vi "Measure H3611i Range.vi"(8 "error in (no error)":errorcluster, 11 "H3611i Actor in":refnum<class "H3611i Actor.lvclass">) -> (0 "error out":errorcluster, 2 "uWave Range(m)":dbl, 3 "H3611i Actor out":refnum<class "H3611i Actor.lvclass">)   [LabVIEW 2018, in "H3611i.lvlib" / "H3611i Actor.lvclass"]
uses:
  H3611i Actor.lvclass
  Datalogger Actor/Data Record Control.ctl
  H3611i Actor.lvclass/H3611i Actor.ctl
  Datalogger Actor/Datalogger Actor.lvclass
panel:
  in  "Data Record":T1
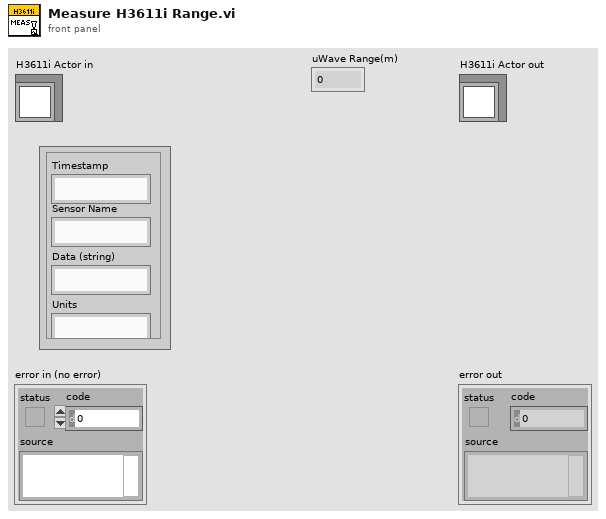
[diagram p1: front panel]
types:
  T1 = typedef "Datalogger.lvlib/Datalogger Actor.lvclass/Data Record Control.ctl" = cluster{"Timestamp":string, "Sensor Name":string, "Data (string)":string, "Units":string}
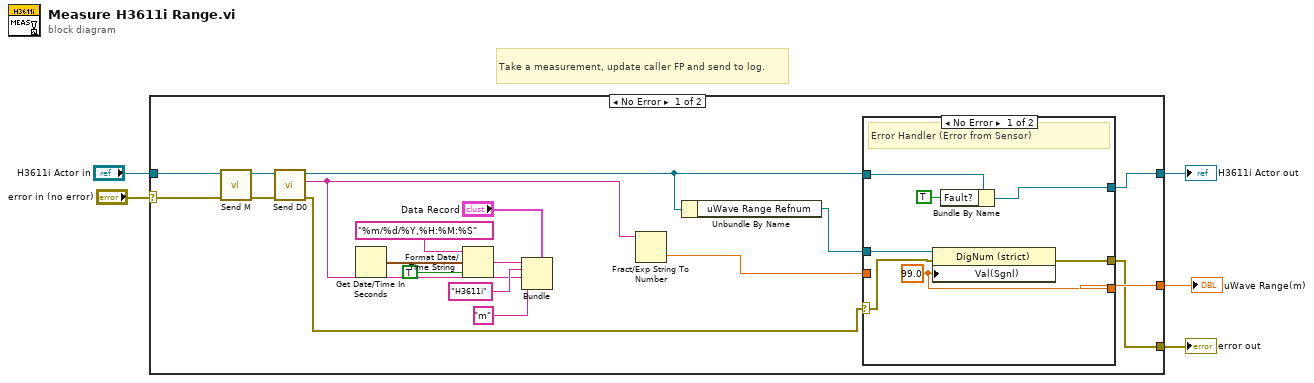
[diagram p0: block diagram]
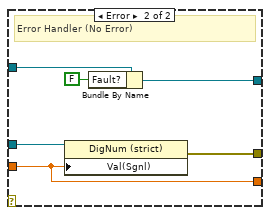
[diagram p2: hidden frame]
diagram:
  # "Take a measurement, update caller FP and send to log."
  n1 = case shown="No Error" "error in (no error)" {
    selector: "error in (no error)" -> [w22 w39]
    tunnel: [w6 w39] -> w4
    tunnel: [w8 w38] -> w2
    tunnel: "H3611i Actor in" -> [w21 w38]
    tunnel: [w11 _] -> w1
    frame No Error {
      n2 = call "Send M.vi"("error in (no error)"=w22, "H3611i Actor in"=w21) -> ("error out"=w23:errorcluster, "H3611i Actor out"=w24:refnum<class "H3611i Actor.lvclass">)  [unwired: 8 in]
      n3 = call "Send D0.vi"("error in (no error)"=w23, "H3611i Actor in"=w24) -> ("error out"=w7:errorcluster, "Range"=w15:string, "H3611i Actor out"=w10:refnum<class "H3611i Actor.lvclass">)  [unwired: 7 in]
      n4 = Get Date/Time In Seconds() -> (seconds since 1Jan1904=w19:timestamp)
      n5 = Format Date/Time String(time format string (%c)="%m/%d/%Y,%H:%M:%S", seconds (now)=w19, UTC format=TRUE) -> (date/time string=w17:string)
      n6 = Bundle(cluster="Data Record", "Timestamp"=w17, "Sensor Name"="H3611i" ("time format string (%c)"), "Data (string)"=w15, "Units"="m" ("time format string (%c)")) -> ()  [unwired: 1 out]
      n7 = Fract/Exp String To Number(string=w15) -> (number=w12:dbl)  [unwired: 3 in, 1 out]
      n8 = Unbundle By Name(w10) -> ("uWave Range Refnum"=w9:refnum<vi>)
      n9 = case shown="No Error" w7 {
        selector: w7 -> [w25 _]
        tunnel: w9 -> [w28 w37]
        tunnel: w12 -> [_ w32]
        tunnel: [w27 w36] -> w6
        tunnel: w10 -> [w31 w35]
        tunnel: [w30 w33] -> w8
        tunnel: [w26 w32] -> w11
        frame No Error {
          w26 = 99.0 ("Value (Signaling)")
          # "Error Handler (Error from Sensor)"
          n10 = property class="DigNum (strict)"(reference=w28, error in=w25, "Val(Sgnl)"=w26) -> (error out=w27:errorcluster)  [unwired: 1 out]
          n11 = Bundle By Name(cluster=w31, "Fault?"=TRUE) -> (w30:refnum<class "H3611i Actor.lvclass">)
        }
        frame Error {
          # "Error Handler (No Error)"
          n12 = property class="DigNum (strict)"(reference=w37, "Val(Sgnl)"=w32) -> (error out=w36:errorcluster)  [unwired: 1 in, 1 out]
          n13 = Bundle By Name(cluster=w35, "Fault?"=FALSE) -> (w33:refnum<class "H3611i Actor.lvclass">)
        }
      }
    }
    frame Error {
    }
  }
  "error out" <- w4
  "H3611i Actor out" <- w2
  "uWave Range(m)" <- w1
